vi "Thread.Get Processor.vi"(11 "Thread in":refnum<class "Thread.lvclass">) -> (2 "Processor":i32, 3 "Thread out":refnum<class "Thread.lvclass">)   [LabVIEW 2017, in "Thread.lvclass"]
uses:
  Thread.lvclass
  Thread.lvclass/Thread.ctl
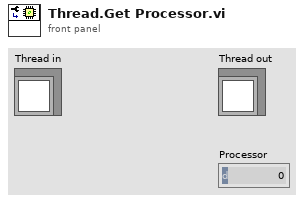
[diagram p1: front panel]
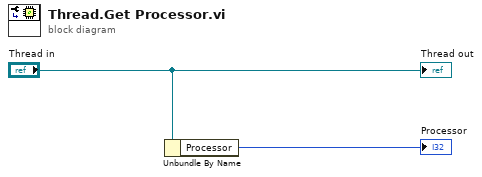
[diagram p0: block diagram]
diagram:
  n1 = Unbundle By Name("Thread in") -> ("Processor"=→"Processor":i32)
  "Thread out" <- "Thread in"
